vi "InitializeMicroscope.vi"(8 "error in (no error)":errorcluster, 11 "Microscope in":refnum<class "Microscope.lvclass">) -> (0 "error out":errorcluster, 3 "Microscope out":refnum<class "Microscope.lvclass">)   [LabVIEW 2012, in "Microscope.lvclass"]
uses:
  classes/Microscope.lvclass
  typedefs/MicroscopeEvent.ctl
  typedefs/ImageEvent.ctl
  classes/Microscope.lvclass/Microscope.ctl
  typedefs/StageEvent.ctl
  variables/GlobalUI.vi
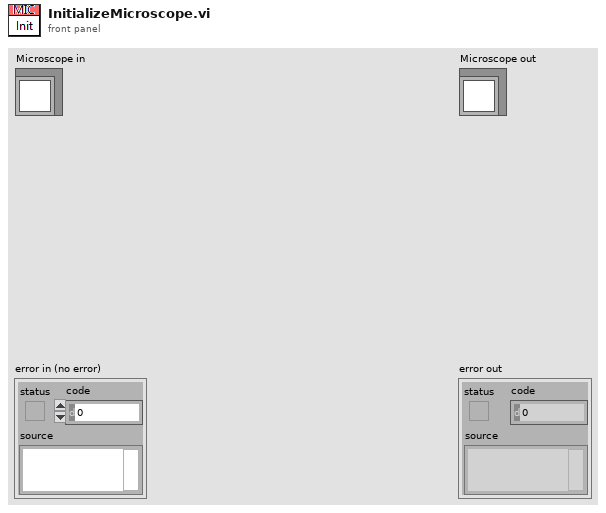
[diagram p1: front panel]
types:
  T1 = typedef "ImageEvent.ctl" = enum16{"i.Wait", "i.Acquire", "i.InitImageData", "i.ReinitImageData", "i.ReinitImageParams", "i.PreAcquire", "i.PostAcquire", "i.ClearData"}
  T2 = typedef "MicroscopeEvent.ctl" = enum16{"M.Wait", "M.RunRotation", "M.Flush", "M.Init", "M.InitStage", "M.InitImageData", "M.ReinitImageData", "M.ReinitImageParams", "M.GetSetParams", "M.InitFastHardware", "M.Pre-Acquire", "M.Acquire", "M.PostAcquire", "M.StopAcquire", "M.SetAcqStatusTrue", "M.SetAcqStatusFalse", "M.ClearImageData", "M.MoveStageDiscrete", "M.MoveStageToTarget1", "M.MoveStageToTarget2", "M.MoveStageToTarget3", "M.OpenShutters", "M.CloseShutters", "M.StartAcquireSequence", "M.ChangeParameters", "M.OpenStokes", "M.OpenPump", "M.RunSW"}
  T3 = typedef "StageEvent.ctl" = enum16{"stage.TimeOut", "stage.FlushData", "stage.GetPosition", "stage.Init", "stage.MoveTo1", "stage.MoveTo2", "stage.MoveTo3", "stage.Stop"}
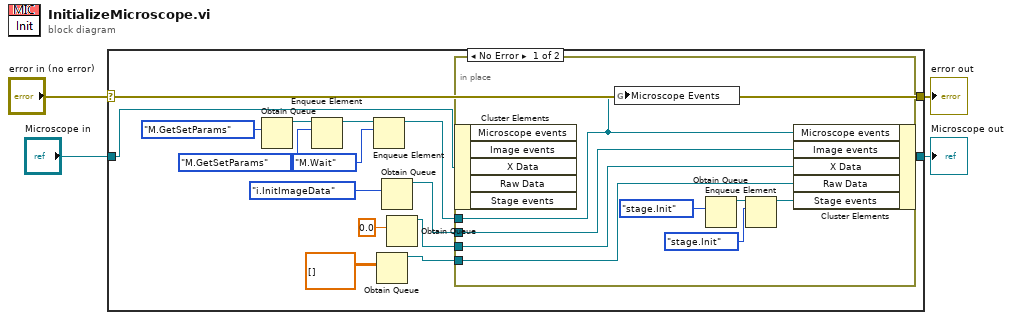
[diagram p0: block diagram]
diagram:
  n1 = case shown="No Error" "error in (no error)" {
    selector: "error in (no error)" -> [w19 w29]
    tunnel: [w19 w29] -> w3
    tunnel: [w11 w28] -> w1
    tunnel: "Microscope in" -> [w13 w28]
    frame No Error {
      n2 = Obtain Queue(element data type=MicroscopeEvent."M.GetSetParams") -> (queue out=w16:refnum<queue>)  [unwired: 4 in, 2 out]
      n3 = Enqueue Element(queue=w16, element=MicroscopeEvent."M.GetSetParams") -> (queue out=w15:refnum<queue>)  [unwired: 2 in, 2 out]
      n4 = Enqueue Element(queue=w15, element=MicroscopeEvent."M.Wait") -> (queue out=w12:refnum<queue>)  [unwired: 2 in, 2 out]
      n5 = Obtain Queue(element data type=dbl[][] [] ("element")) -> (queue out=w6:refnum<queue>)  [unwired: 4 in, 2 out]
      n6 = Obtain Queue(element data type=ImageEvent."i.InitImageData" ("element")) -> (queue out=w8:refnum<queue>)  [unwired: 4 in, 2 out]
      n7 = Obtain Queue(element data type=0.0 ("x")) -> (queue out=w7:refnum<queue>)  [unwired: 4 in, 2 out]
      n8 = in-place {
        in-place-border: w12 -> [w20]
        in-place-border: w8 -> [w26]
        in-place-border: w7 -> [w21]
        in-place-border: w6 -> [w27]
        n9 = in-place-cluster #1(w13) -> ()  [unwired: 5 out]
        n10 = global write "GlobalUI.vi" "Microscope Events"(w20) -> ()
        n11 = Obtain Queue(element data type=StageEvent."stage.Init") -> (queue out=w24:refnum<queue>)  [unwired: 4 in, 2 out]
        n12 = Enqueue Element(queue=w24, element=StageEvent."stage.Init") -> (queue out=w22:refnum<queue>)  [unwired: 2 in, 2 out]
        n13 = in-place-cluster #1("Microscope events"=w20, "Image events"=w26, "X Data"=w21, "Raw Data"=w27, "Stage events"=w22) -> (w11:refnum<class "Microscope.lvclass">)
      }
    }
    frame Error {
    }
  }
  "error out" <- w3
  "Microscope out" <- w1
